vi "ClimbGlobal.vi"() -> ()   [LabVIEW 2023]
panel:
  out "Debug_Cancel":i32
  out "Debug_Reach":i32
  out "Debug_Pull":i32
  out "Debug_DecCount":i32
  out "Debug_IncCount":i32
  in  "PullLimit":bool
  in  "ReachLimit":bool
  in  "SensorPosition":dbl
  in  "ClimbMotorDmd":dbl
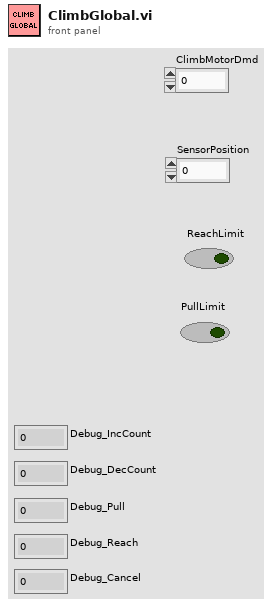
[diagram p1: front panel]
diagram:
